vi "DebugToConsole.vi"(8 "error in (no error)":errorcluster, 11 "String":string) -> (0 "error out":errorcluster)   [LabVIEW 2017]
panel:
  out "error out 2":errorcluster
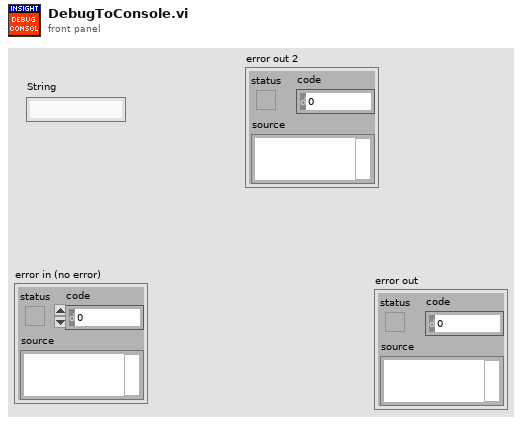
[diagram p1: front panel]
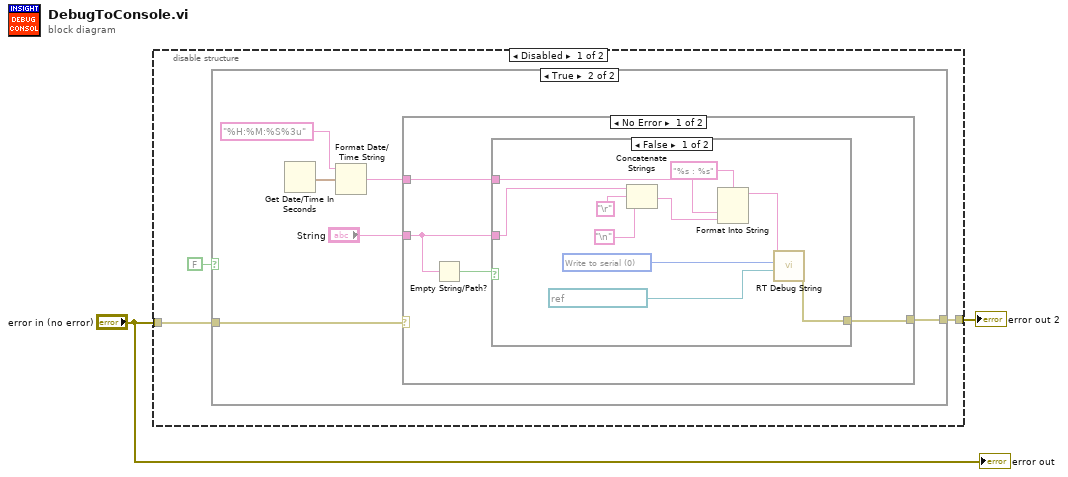
[diagram p0: block diagram]
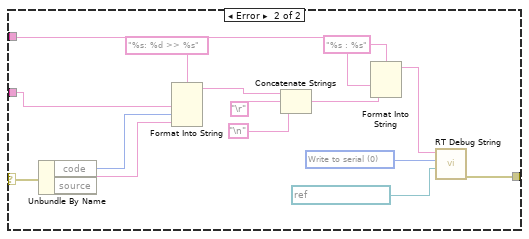
[diagram p4: hidden frame]
diagram:
  n1 = disable-structure shown="Disabled" {
    disable-tunnel: [w5 _] -> w2
    disable-tunnel: "error in (no error)" -> [w4 _]
    frame Disabled {
      n2 = case shown="True" FALSE {
        tunnel: [_ w10] -> w5
        tunnel: w4 -> [_ w9]
        frame False {
        }
        frame True {
          n3 = Get Date/Time In Seconds() -> (seconds since 1Jan1904=w8:timestamp)
          n4 = Format Date/Time String(time format string (%c)="%H:%M:%S%3u", seconds (now)=w8) -> (date/time string=w7:string)  [unwired: 1 in]
          n5 = case shown="No Error" w9 {
            selector: w9 -> [_ w30]
            tunnel: "String" -> [w14 w38]
            tunnel: [w13 w36] -> w10
            tunnel: w7 -> [w12 w28]
            frame No Error {
              n6 = Empty String/Path?(string/path=w14) -> (empty?=w15:bool)
              n7 = case shown="False" w15 {
                tunnel: w14 -> [w20 _]
                tunnel: [w23 _] -> w13
                tunnel: w12 -> [w17 _]
                frame False {
                  w25 = u16 0 items=["Write to serial", "Write to monitor"] ("Interface")
                  n8 = Concatenate Strings(w20, "\r", "\n") -> (w18:string)
                  n9 = Format Into String(format string="%s : %s", w17, w18) -> (resulting string=w16:string)  [unwired: 2 in, 1 out]
                  n10 = call <vilib>:"RT Debug String.vi"("VISA resource name"=refnum<visa-resource-name> "ASRL1::INSTR", "Interface"=w25, "String to write"=w16) -> ("error out"=w23:errorcluster)  [unwired: 8 in]
                }
                frame True {
                }
              }
            }
            frame Error {
              w40 = u16 0 items=["Write to serial", "Write to monitor"] ("Interface")
              n11 = Unbundle By Name(w30) -> ("code"=w32:i32, "source"=w31:string)
              n12 = Format Into String(format string="%s: %d >> %s", w38, w32, w31) -> (resulting string=w37:string)  [unwired: 2 in, 1 out]
              n13 = Concatenate Strings(w37, "\r", "\n") -> (w27:string)
              n14 = Format Into String(format string="%s : %s", w28, w27) -> (resulting string=w26:string)  [unwired: 2 in, 1 out]
              n15 = call <vilib>:"RT Debug String.vi"("VISA resource name"=refnum<visa-resource-name> "ASRL1::INSTR", "Interface"=w40, "String to write"=w26) -> ("error out"=w36:errorcluster)  [unwired: 8 in]
            }
          }
        }
      }
    }
    frame Enabled {
    }
  }
  "error out 2" <- w2
  "error out" <- "error in (no error)"
